vi "Get_RF_scale.vi"(9 "rho-":dbl[](array[numeric]), 10 "rho0":dbl[](array[numeric]), 11 "rho+":dbl[](array[numeric])) -> (2 "I-  index out":dbl, 3 "I+ index out":dbl)   [LabVIEW 2018]
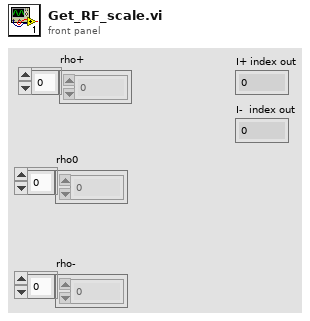
[diagram p1: front panel]
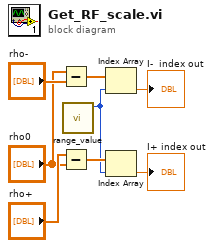
[diagram p0: block diagram]
diagram:
  n1 = Subtract(x="rho0", y="rho-") -> (x-y=w5:dbl[])
  n2 = Subtract(x="rho+", y="rho0") -> (x-y=w4:dbl[])
  n3 = call "range_value.vi"() -> ("Center"=w2:i32)  [unwired: 10 in, 1 out]
  n4 = Index Array(array=w5, index=w2) -> (element=→"I-  index out":dbl)
  n5 = Index Array(array=w4, index=w2) -> (element=→"I+ index out":dbl)
